vi "Connect_Func.vi"(8 "error in (no error)":errorcluster, 11 "Data Cluster in":T1) -> (0 "error out":errorcluster, 2 "Connected":bool, 3 "Data Cluster out":T1)   [LabVIEW 2017, in "FingerPrintMânager.lvlib"]
uses:
  Module Data--cluster.ctl
  <vilib>/Instr/_visa.llb/VISA Configure Serial Port (Instr).vi
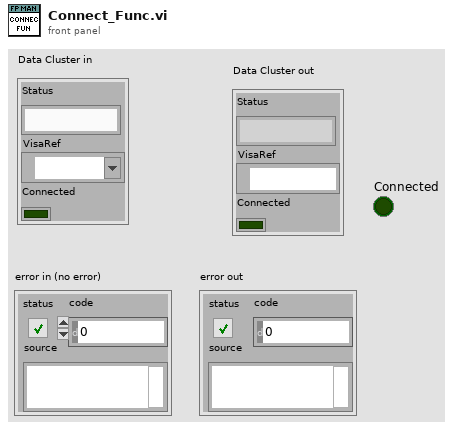
[diagram p1: front panel]
types:
  T1 = typedef "FingerPrintMânager.lvlib/Module Data--cluster.ctl" = cluster{"Status":string, "VisaRef":refnum<visa-resource-name>, "Connected":bool}
  T2 = cluster{"baud rate":u32, "data bits":u16, "parity":enum16{"None", "Odd", "Even", "Mark", "Space"}, "stop bits":u16, "flow control":u16}
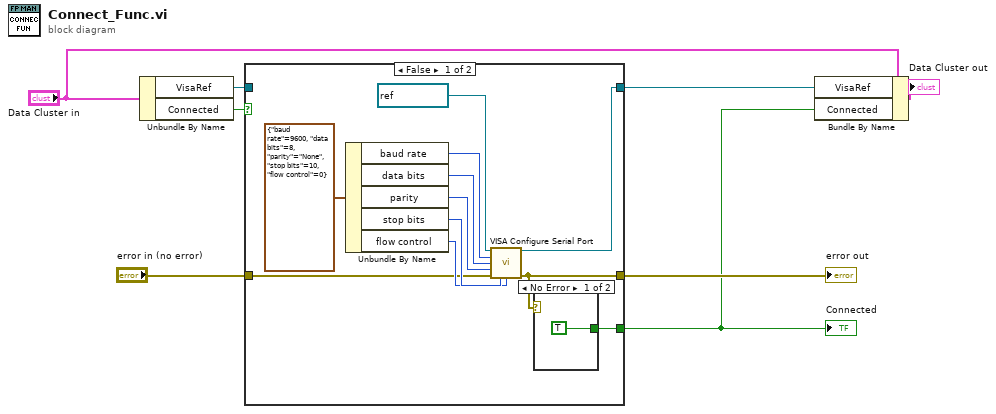
[diagram p0: block diagram]
diagram:
  n1 = Unbundle By Name("Data Cluster in") -> ("VisaRef"=w3:refnum<visa-resource-name>, "Connected"=w2:bool)
  n2 = case shown="False" w2 {
    selector: w2 -> [_ w21]
    tunnel: "error in (no error)" -> [w13 w23]
    tunnel: [w11 w23] -> w6
    tunnel: [w12 w22] -> w8
    tunnel: w3 -> [_ w22]
    tunnel: [w9 w21] -> w1
    frame False {
      n3 = Unbundle By Name(T2 {"baud rate"=9600, "data bits"=8, "parity"=enum."None", "stop bits"=10, "flow control"=0} ("Serial Settings 2")) -> ("baud rate"=w18:u32, "data bits"=w17:u16, "parity"=w16:enum16{"None", "Odd", "Even", "Mark", "Space"}, "stop bits"=w15:u16, "flow control"=w14:u16)
      n4 = call-poly "VISA Configure Serial Port"("VISA resource name"=refnum<visa-resource-name> "COM1", "baud rate (9600)"=w18, "data bits (8)"=w17, "parity (0:none)"=w16, "error in (no error)"=w13, "stop bits (10: 1 bit)"=w15, "flow control (0:none)"=w14) -> ("VISA resource name out"=w12:refnum<visa-resource-name>, "error out"=w11:errorcluster)  [unwired: 2 in, 5 out]
      n5 = case shown="No Error" w11 {
        tunnel: [TRUE _] -> w9
        frame No Error {
        }
        frame Error {
        }
      }
    }
    frame True {
    }
  }
  "error out" <- w6
  "Connected" <- w1
  n6 = Bundle By Name(cluster="Data Cluster in", "VisaRef"=w8, "Connected"=w1) -> (→"Data Cluster out":T1)
